vi "Configure Jitter Analysis.vi"(5 "Enable Jitter Spectrum (F: Disable)":bool, 6 "Enable Jitter Trend (F: Disable)":bool, 7 "Enable Jitter Histogram (F: Disable)":bool, 8 "error in (no error)":errorcluster, 9 "Jitter Source (1: Measurement1)":i32(ring)=1 items=["Measurement 1"=1, "Measurement 2"=2, "Measurement 3"=3, "Measurement 4"=4, "Measurement 5"=5, "Measurement 6"=6, "Measurement 7"=7, "Measurement 8"=8, "Measurement 9"=9, "Measurement 10"=10], 10 "Enable Jitter Analysis (T: Enable)":bool=TRUE, 11 "VISA resource name":refnum<visa-resource-name>) -> (0 "error out":errorcluster, 3 "VISA resource name out":refnum<visa-resource-name>)   [LabVIEW 2015, in "Agilent 2000 3000 X-Series.lvlib"]
doc: "Enables/disables the jitter analysis feature and specifies the measurement to be analyzed. The jitter measurement must be configured and enabled prior to selecting it. Enables/disables Jitter Histogram, Spectrum and Trend features.\n\n<b>Note:</b>\nThis VI is specific to the 6000-X Series oscilloscopes. These features are not available on other models."
uses:
  Agilent 2000 3000 X-Series.lvlib
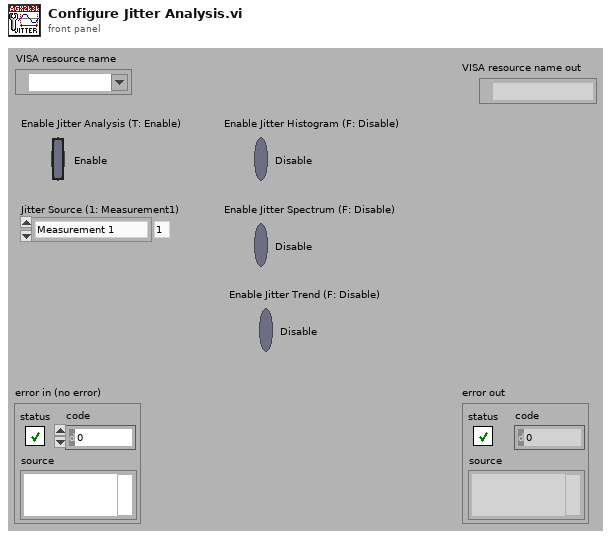
[diagram p1: front panel]
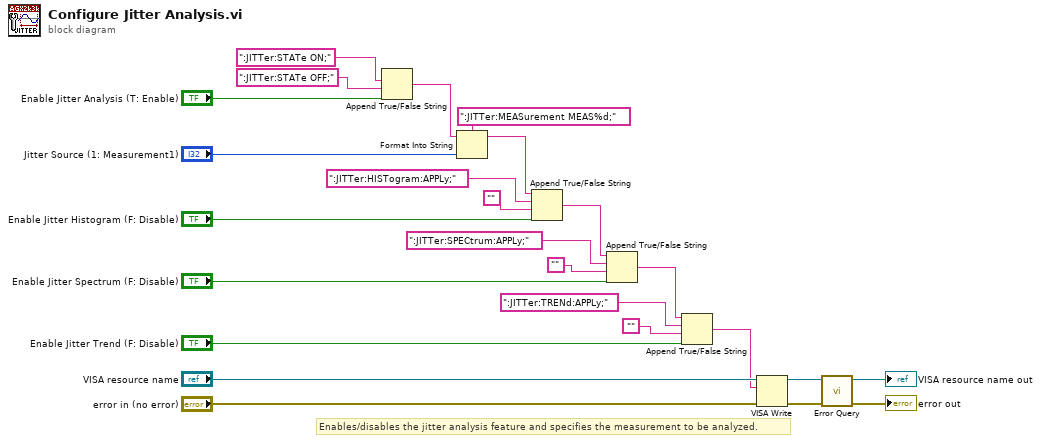
[diagram p0: block diagram]
diagram:
  # "Enables/disables the jitter analysis feature and specifies the measurement to be analyzed."
  n1 = Append True/False String(1:"Enable Jitter Analysis (T: Enable)", 2:":JITTer:STATe OFF;", 3:":JITTer:STATe ON;") -> (0:w22:string)  [unwired: 1 in]
  n2 = Format Into String(format string=":JITTer:MEASurement MEAS%d;", initial string=w22, "Jitter Source (1: Measurement1)") -> (resulting string=w19:string)  [unwired: 1 in, 1 out]
  n3 = Append True/False String(1:"Enable Jitter Histogram (F: Disable)", 2:"", 3:":JITTer:HISTogram:APPLy;", 4:w19) -> (0:w6:string)
  n4 = Append True/False String(1:"Enable Jitter Spectrum (F: Disable)", 2:"", 3:":JITTer:SPECtrum:APPLy;", 4:w6) -> (0:w13:string)
  n5 = Append True/False String(1:"Enable Jitter Trend (F: Disable)", 2:"", 3:":JITTer:TRENd:APPLy;", 4:w13) -> (0:w5:string)
  n6 = VISA Write(VISA resource name="VISA resource name", write buffer=w5, error in (no error)="error in (no error)") -> (VISA resource name out=w4:refnum<visa-resource-name>, error out=w3:errorcluster)  [unwired: 1 out]
  n7 = call "Error Query.vi"("error in (no error)"=w3, "VISA resource name"=w4) -> ("error out"=→"error out":errorcluster, "VISA resource name out"=→"VISA resource name out":refnum<visa-resource-name>)  [unwired: 6 in, 2 out]
